vi "Check for Custom Changes.vi"(8 "error in (no error)":errorcluster, 10 "Message Class":refnum<vi>) -> (0 "error out":errorcluster)   [LabVIEW 2023, in "Message Maker.lvclass"]
doc: "Calculates the checksum for the message's items and compares it to the stored value. If a change is detected the user is asked if they'd like to blow away these custom changes\n\nAuthor: Derek Trepanier\nCopyright: MGI 2015"
uses:
  Message Maker.lvclass
  Message Maker.lvclass/Message Maker.ctl
  <vilib>/ErrorRing/Error Ring.xnode
  <vilib>/Utility/error.llb/Error Cluster From Error Code.vi
panel:
  out "Array":string[](array[string])
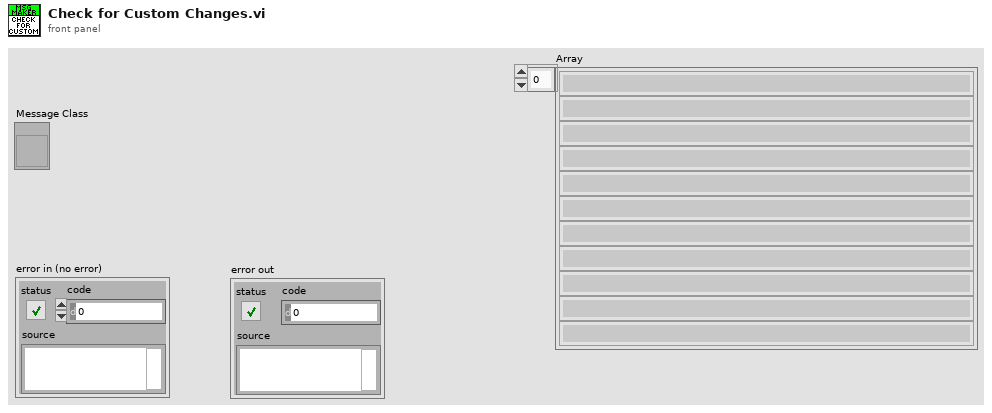
[diagram p1: front panel]
types:
  T1 = enum16{"Left Button", "Center Button", "Right Button", "Window Close"}
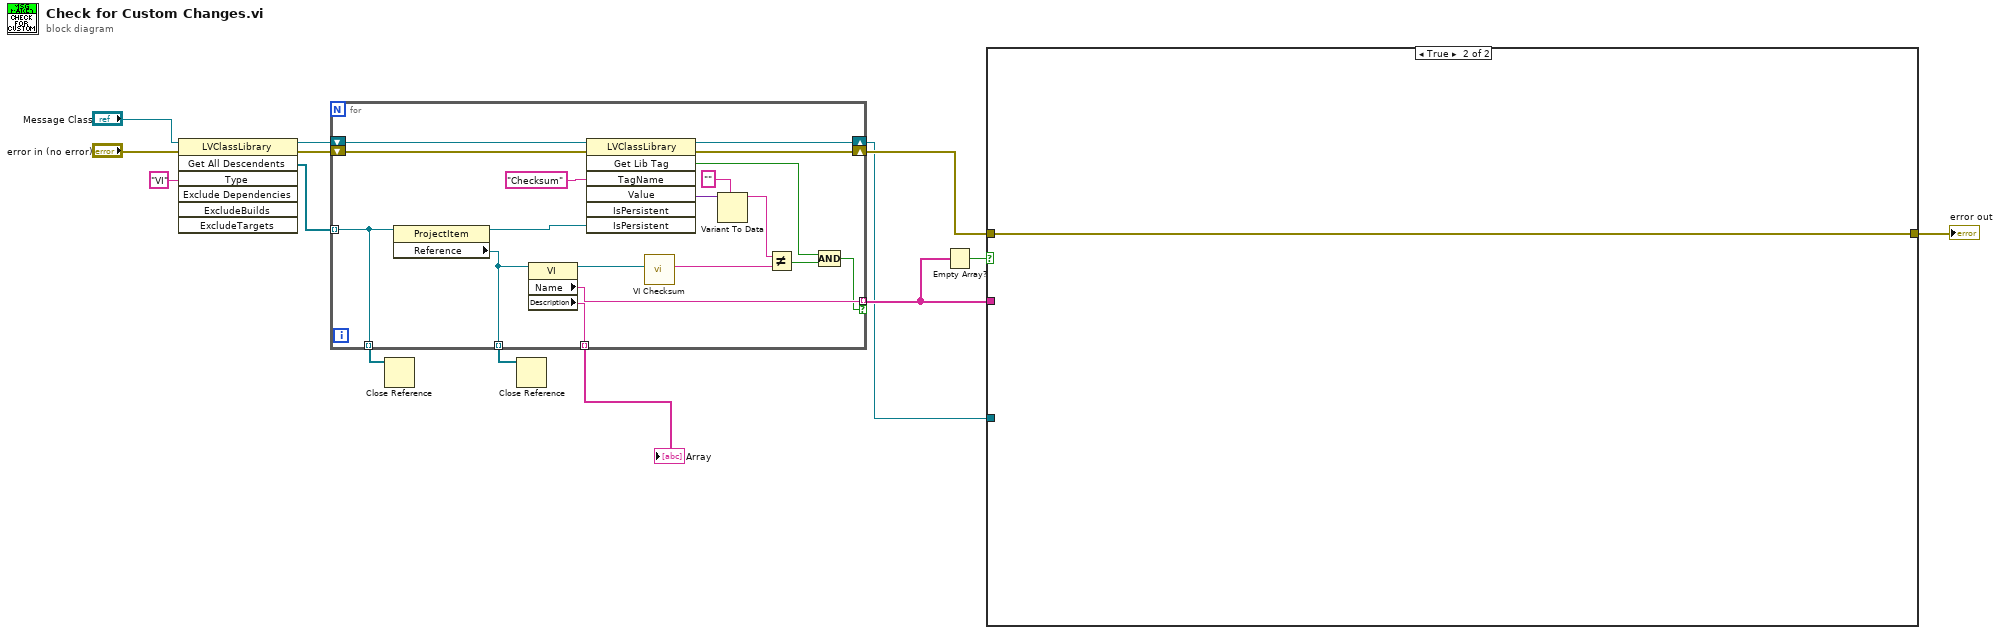
[diagram p0: block diagram]
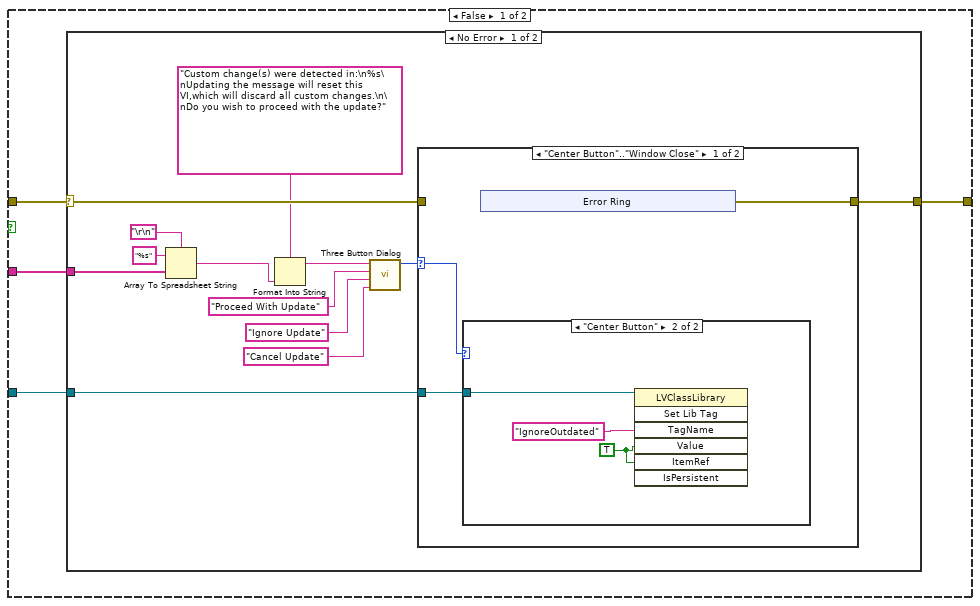
[diagram p2: hidden frame]
diagram:
  n1 = invoke class="LVClassLibrary" method="Get All Descendents"(reference="Message Class", error in="error in (no error)", "Type"="VI") -> (reference out=w12:refnum<vi>, error out=w11:errorcluster, "All Descendents"=w10:refnum<vi>[])  [unwired: 4 in, 4 out]
  n2 = for {
    tunnel: w10 -> [w16] mode=indexing
    shift-right: [w31] -> w2
    shift-left: w12 -> [w32]
    shift-right: [w29] -> w14
    shift-left: w11 -> [w30]
    tunnel: [w19] -> w7 mode=indexing if=w18
    tunnel: [w17] -> w4 mode=indexing
    tunnel: [w16] -> w3 mode=indexing
    tunnel: [w15] -> w1 mode=indexing
    n3 = property class="ProjectItem"(reference=w16) -> (reference out=w22:refnum<vi>, "Reference"=w17:refnum<vi>)  [unwired: 1 in, 1 out]
    n4 = property class="VI"(reference=w17) -> (reference out=w20:refnum<vi>, "Name"=w19:string, "Description"=w15:string)  [unwired: 1 in, 1 out]
    n5 = invoke class="LVClassLibrary" method="Get Lib Tag"(reference=w32, error in=w30, "TagName"="Checksum" ("Tag Name"), "IsPersistent"=w22) -> (reference out=w31:refnum<vi>, error out=w29:errorcluster, "GetTag"=w23:bool, "Value"=w28:variant)  [unwired: 3 in, 3 out]
    n6 = call "VI Checksum.vi"("VI"=w20) -> ("VI Checksum"=w25:string)  [unwired: 10 in]
    n7 = Variant To Data(type="", Variant=w28) -> (data=w26:string)  [unwired: 1 in, 1 out]
    n8 = Not Equal?(x=w26, y=w25) -> (x != y?=w24:bool)
    n9 = Compound Arithmetic op=AND(w23, w24) -> (w18:bool)
  }
  "Array" <- w1
  n10 = Close Reference(reference=w3) -> ()  [unwired: 1 in, 1 out]
  n11 = Close Reference(reference=w4) -> ()  [unwired: 1 in, 1 out]
  n12 = Empty Array?(array=w7) -> (empty?=w6:bool)
  n13 = case shown="True" w6 {
    tunnel: w14 -> [w34 w62]
    tunnel: w7 -> [w36 _]
    tunnel: [w35 w62] -> w5
    tunnel: w2 -> [w33 _]
    frame False {
      n14 = case shown="No Error" w34 {
        selector: w34 -> [w43 w61]
        tunnel: w36 -> [w49 _]
        tunnel: [w44 w61] -> w35
        tunnel: w33 -> [w37 _]
        frame No Error {
          n15 = Array To Spreadsheet String(delimiter (Tab)="\r\n", array=w49, 3:"%s" ("format string")) -> (spreadsheet string=w41:string)
          n16 = Format Into String(format string="Custom change(s) were detected in:\n%s\nUpdating the message will reset this VI,which will discard all custom changes.\n\nDo you wish to proceed with the update?" ("message"), w41) -> (resulting string=w46:string)  [unwired: 2 in, 1 out]
          n17 = call <vilib>:"Three Button Dialog.vi"("Right Button Text (\"Cancel\")"="Cancel Update" ("F button name (\"Cancel\")"), "Center Button Text (\"No\")"="Ignore Update" ("T button name (\"OK\")"), "Left Button Text (\"Yes\")"="Proceed With Update" ("T button name (\"OK\")"), "message"=w46) -> ("Which Button?"=w45:T1)  [unwired: 7 in]
          n18 = case shown="\"Center Button\"..\"Window Close\"" w45 {
            selector: w45 -> [w50 _]
            tunnel: [w52 w60] -> w44
            tunnel: w43 -> [_ w60]
            tunnel: w37 -> [w51 _]
            frame "Center Button".."Window Close" {
              n19 = case shown="\"Center Button\"" w50 {
                tunnel: w51 -> [_ w55]
                frame Default {
                }
                frame "Center Button" {
                  w54 = TRUE
                  n20 = invoke class="LVClassLibrary" method="Set Lib Tag"(reference=w55, "TagName"="IgnoreOutdated" ("Tag Name"), "Value"=w54, "ItemRef"=w54) -> ()  [unwired: 3 in, 7 out]
                }
              }
              n21 = xnode "Error Ring"() -> ("error out"=w52:errorcluster)
            }
            frame "Left Button" {
            }
          }
        }
        frame Error {
        }
      }
    }
    frame True {
    }
  }
  "error out" <- w5
